vi "x410_test_fpga_simple.vi"() -> ()   [LabVIEW 2025]
doc: "this VI is the top level of the FPGA.\n\nsubVIs placed at this level:\nmust have fixed-sized arrays.\ncontaining a class input (control) must NOT be left unconnected.\n\nconditional symbols supported for ease-of-use in building variations of the image are documented in a comment section and should be kept up-to-date."
uses:
  Aqc_loop_states.ctl
  <instrlib>/_niInstr/DSP/v1/Shared/Public/IQ Gain.ctl
  FPGA/DataMode.ctl
  <vilib>/Platform/TimedLoop/XDataNode/timing_clust.ctl
  <vilib>/Platform/TimedLoop/XDataNode/nitl_modes.ctl
  <vilib>/Platform/TimedLoop/XDataNode/wakeup.ctl
  <vilib>/rvi/Emulation/niFpgaSctlEmulationGetInTimedLoop.vi
  <vilib>/rvi/Emulation/niFpgaEmulationReportErrorSimple.vi
  <vilib>/rvi/Emulation/niFpgaGetClockAttributes.vi
  <vilib>/rvi/Emulation/niFpgaCriticalErrorInLSC.vi
  <vilib>/rvi/Emulation/niFpgaEmulationIsFPGAContextNoSignature.vi
  <vilib>/rvi/DataTransferAndStorage/Container/Common/niFpgaContainerGetUniqueNameForEmu.vi
  <vilib>/rvi/Memory/Memory_Emulation/niFpgaMemoryEmulationCacheClearOnFirstRun.vi
  <vilib>/rvi/Memory/Memory_Emulation/nirvimemoryEmulationManagerCache_MakeExclusive.vi
  <vilib>/rvi/Memory/Memory_Emulation/niFpgaMemoryEmulationValidateCache.vi
  <vilib>/rvi/Memory/Memory_Emulation/nirvimemoryEmulationManagerCache_InsertValue.vi
  <vilib>/Utility/error.llb/Clear Errors.vi
  <vilib>/rvi/Memory/Memory_Emulation/nirvimemoryEmulationManagerCache_ReleaseExclusive.vi
  <vilib>/rvi/Memory/Memory_Emulation/nirvimemoryEmulationManagerCache_GetValue.vi
  <vilib>/rvi/Memory/Memory_Emulation/nirvimemoryEmulationManagerCache_SetValue.vi
  <vilib>/rvi/Emulation/niFpgaProcessEmulError.vi
  <vilib>/rvi/errors/niFpgaSetErrorForExecOnDevCompSimple.vi
  <vilib>/rvi/eio/common/nirviEmuReportErrorAndStop.vi
  <vilib>/rvi/FIFO/Fifo_Resource/nirvififoEmulationSetSize.vi
  <vilib>/rvi/FIFO/Fifo_Resource/nirviFifoEmulationQueueMgr.vi
  <instcachedir>/0/nirviFifoEmulationQueueMgr_E5CAEC123FF24DC58D834DCA3CDAA9B5.lvgen/nirviFifoEmulationQueueMgr_E5CAEC123FF24DC58D834DCA3CDAA9B5_017.vi
  <vilib>/rvi/FIFO/Fifo_Resource/nirvififoEmulationCreateLock.vi
  <vilib>/rvi/FIFO/Fifo_Resource/nirvififoEmulationObtainLock.vi
  <vilib>/rvi/FIFO/Fifo_Resource/nirvififoEmulationReleaseLock.vi
  <vilib>/rvi/occurrence/nirviWaitOnOccurrenceBase.vi
  <vilib>/rvi/errors/nirviReportUnexpectedCaseInternalError.vi
  <vilib>/rvi/errors/nirviReportUnexpectedCaseInternalError (U32).vi
  <instcachedir>/0/nirviFifoEmulationQueueMgr_E5CAEC123FF24DC58D834DCA3CDAA9B5.lvgen/nirviFifoEmulationQueueMgr_E5CAEC123FF24DC58D834DCA3CDAA9B5_016.vi
  <vilib>/rvi/FIFO/Fifo_Resource/nirvififoEmulationDetermineInputValidOut.vi
  <vilib>/rvi/interface/RandomDataEmulation/nirviRandomDataMultiElementFPGAFIFO.vi
  <instcachedir>/0/nirviRandomDataMultiElementFPGAFIFO_BE2FF10D3D6E420AB0291A02835C249E.lvgen/nirviRandomDataMultiElementFPGAFIFO_BE2FF10D3D6E420AB0291A02835C249E_001.vi
  <vilib>/rvi/interface/RandomDataEmulation/niFpgaRandomDataHandleErrors.vi
  <vilib>/Platform/TimedLoop/XDataNode/XDataNode.xnode
  <vilib>/rvi/DataTransferAndStorage/Container/XNode/niFpgaContainer.xnode
  <vilib>/rvi/DataTransferAndStorage/Register/Emulation/niFpgaRegisterEmulation.vi
  <vilib>/rvi/FIFO/Fifo_Resource/nirvififoEmulationRead.vi
  <vilib>/rvi/FIFO/Fifo_Resource/nirvififoEmulationWrite.vi
  <vilib>/rvi/interface/RandomDataEmulation/nirviRandomDataFpgaMultiElementTemplate.vi
  <vilib>/Platform/TimedLoop/XDataNode/XDNodeRunTimeDep.lvlib
  <instrlib>/niUSRP/Reference FPGA/Tx Core/niUSRP Tx Core v1 FPGA.lvclass
  <instrlib>/_niInstr/DSP/v1/Shared/niInstr DSP v1 Shared.lvlib
panel:
  in  "Host scale":u16
  in  "simulated phase":fxp<+,64,64>
  in  "Mode":T1
  in  "gain":T2={"gain I"=1.0, "gain Q"=1.0}
  out "loop states":T3
  in  "Record length":u16=4000 caption="Samples Per Trigger" min=1 step=1
  in  "Trigger Acquisition":bool
  in  "Acquisition running":bool
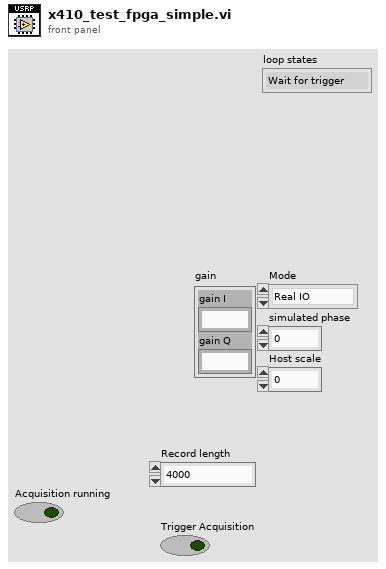
[diagram p1: front panel]
types:
  T1 = typedef "DataMode.ctl" = enum16{"Real IO", "Simulated"}
  T2 = typedef "niInstr DSP v1 Shared.lvlib/IQ Gain.ctl" = cluster{"gain I":fxp<+/-,24,3>, "gain Q":fxp<+/-,24,3>}
  T3 = typedef "Aqc_loop_states.ctl" = enum8{"Wait for trigger", "Acquisition", "Send record length", "Wait for output", "Quiet period"}
  T4 = typedef "XDNodeRunTimeDep.lvlib/timing_clust.ctl" = cluster{"Expected End [f-1]":u64, "Actual End [f-1]":u64, "Finished Late? [f-1]":bool, "Expected End [i-1]":u64, "Actual End [i-1]":u64, "Finished Late? [i-1]":bool, "Expected Start [i]":u64, "Actual Start [i]":u64, "Expected Start [f]":u64, "Actual Start [f]":u64, "Source Name":string, "Structure Name":string, "Period":i64, "Deadline":i64, "Offset":i64, "Start":i64, "Priority":i32, "Timeout":i32, "Mode":T5, "Wakeup Reason":T6, "Error":errorcluster, "Source Type":string, "Secondary Source Type":string, "Global End Time":u64, "Global Start Time":u64, "Frame Duration":u64, "Iteration Duration":u64, "Assigned CPU":i32, "I/O Scan Engine Mode":u32}
  T5 = typedef "XDNodeRunTimeDep.lvlib/nitl_modes.ctl" = enum32{"No Change", "Process missed periods, maintain original phase", "Discard missed periods, maintain original phase", "Process missed periods, ignore original phase", "Discard missed periods, ignore original phase"}
  T6 = typedef "XDNodeRunTimeDep.lvlib/wakeup.ctl" = enum32{"Normal", "Aborted", "Asynchronous wakeup", "Timing source error", "Timed loop error", "Timeout"}
  T7 = cluster{"I":fxp<+/-,18,1>, "Q":fxp<+/-,18,1>, "overflow":bool}[]
  T8 = typedef "niInstr DSP v1 Shared.lvlib/IQ Data.ctl" = cluster{"I":fxp<+/-,18,1>, "Q":fxp<+/-,18,1>, "overflow":bool}
  T9 = typedef "Array-18bit-8element.ctl" = fxp<+/-,18,1>[]
  T10 = cluster{"I":fxp<+/-,18,1>, "Q":fxp<+/-,18,1>, "overflow":bool}
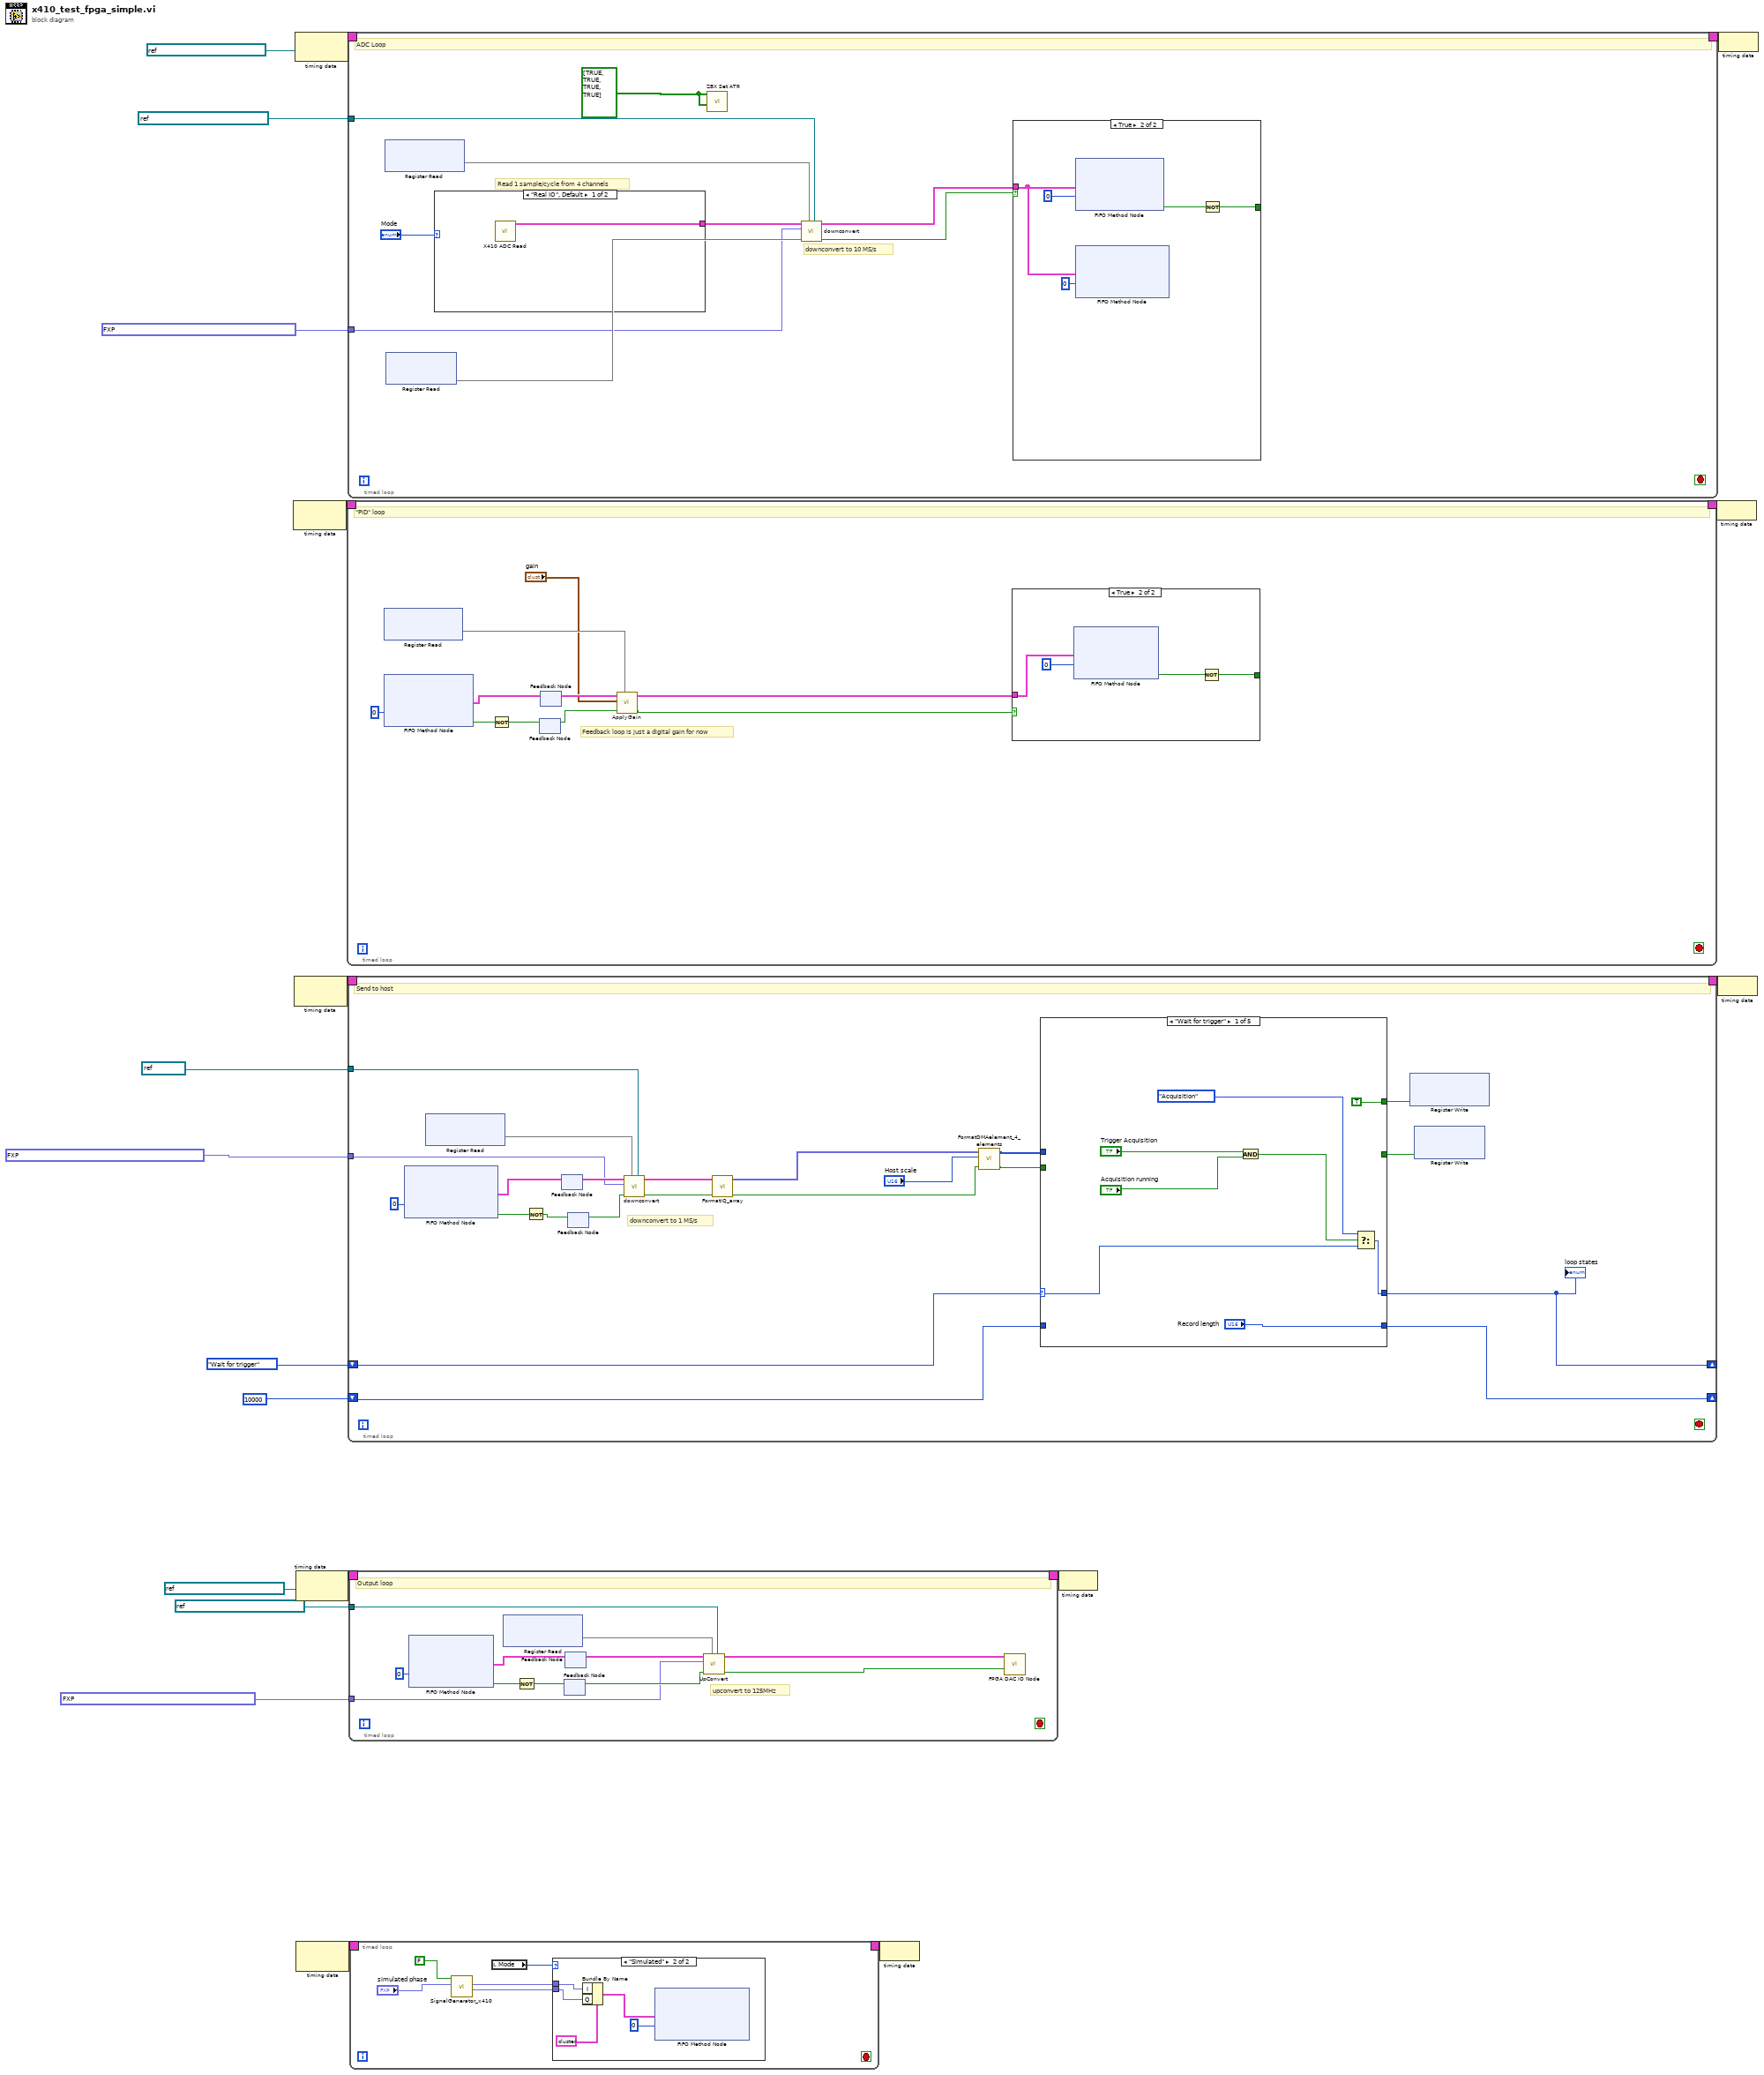
[diagram p0: block diagram]
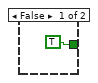
[diagram p3: hidden frame]
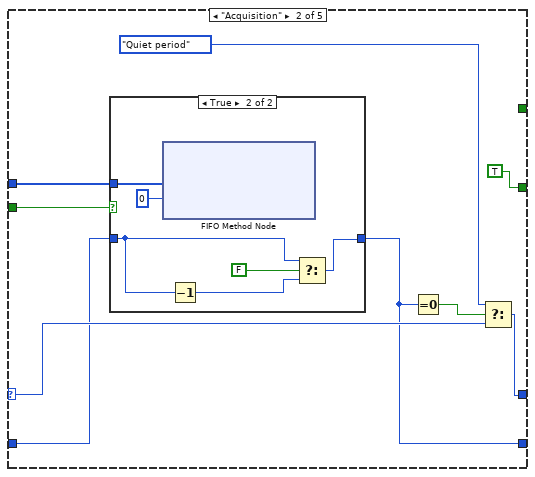
[diagram p4: hidden frame]
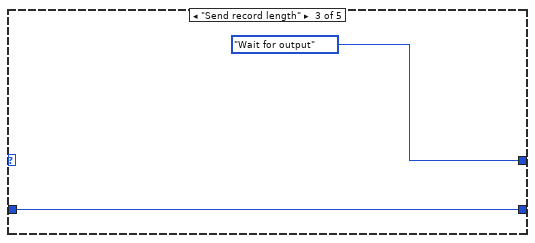
[diagram p6: hidden frame]
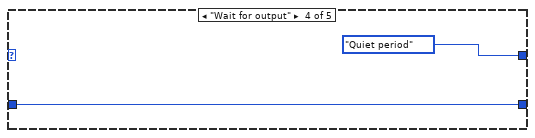
[diagram p7: hidden frame]
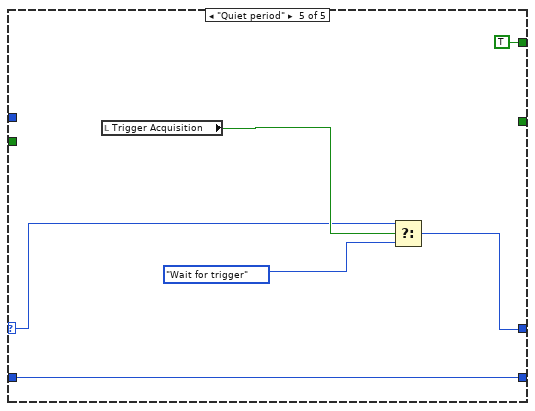
[diagram p8: hidden frame]
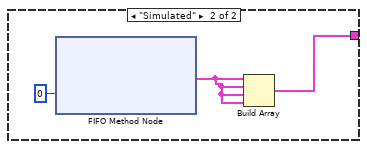
[diagram p9: hidden frame]
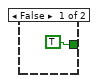
[diagram p10: hidden frame]
diagram:
  n1 = node-c288() -> (w11:T4)  [unwired: 1 in]
  n2 = node-c288() -> (w17:T4)  [unwired: 1 in]
  n3 = node-c288(refnum<k21> "Daughterboard 0\\Data Clock" ("Source Name")) -> (w20:T4)
  n4 = node-c288(refnum<k21> "Daughterboard 0\\Data Clock" ("Source Name")) -> (w7:T4)
  n5 = node-c288() -> (w2:T4)  [unwired: 1 in]
  n6 = timed-loop "Acquisition Loop" {
    timing: w11 -> [_]
    timing-out: [_] -> w10
    stop <- _ stop-if-true
    # "Feedback loop is just a digital gain for now"
    # "\"PID\" loop"
    n7 = xnode "Register Read"() -> ("Data"=w25)  [unwired: 1 in, 1 out]
    n8 = xnode ("FIFO Method Node")("Timeout"=0) -> ("Element"=w29:T7, "Timed Out?"=w30:bool)  [unwired: 1 in, 1 out]
    n9 = Not(x=w30) -> (.not. x?=w27:bool)
    n10 = feedback #1() -> (w26:bool)  [unwired: 1 in]
    n11 = feedback-in #1(w27) -> ()
    n12 = feedback #2() -> (w28:T7)  [unwired: 1 in]
    n13 = feedback-in #2(w29) -> ()
    n14 = call "ApplyGain.vi"("reset"=w25, "input valid"=w26, "gain"="gain", "data in"=w28) -> ("output valid"=w23:bool, "data out"=w22:T8[])  [unwired: 6 in]
    n15 = case shown="True" w23 {
      tunnel: [TRUE ("Timed Out?") w33] -> _
      tunnel: w22 -> [_ w32]
      frame False {
      }
      frame True {
        n16 = xnode ("FIFO Method Node")("Element"=w32, "Timeout"=0) -> ("Timed Out?"=w34:bool)  [unwired: 1 in, 1 out]
        n17 = Not(x=w34) -> (.not. x?=w33:bool)
      }
    }
  }
  n18 = timed-loop "Acquisition Loop" {
    timing: w17 -> [_]
    timing-out: [_] -> w16
    shift-right: [w55] -> _
    shift-left: u16 10000 ("Record length") -> [w53]
    shift-right: [w56] -> _
    shift-left: Aqc_loop_states."Wait for trigger" ("loop states") -> [w54]
    tunnel: refnum<k21> "20MHz" ("clock x2") -> [w44]
    tunnel: fxp<+,48,1> 0.10000000000000142 ("output sample rate") -> [w42]
    stop <- _ stop-if-true
    # "downconvert to 1 MS/s"
    # "Send to host"
    n19 = xnode ("FIFO Method Node")("Timeout"=0) -> ("Element"=w49:T7, "Timed Out?"=w51:bool)  [unwired: 1 in, 1 out]
    n20 = xnode "Register Read"() -> ("Data"=w43)  [unwired: 1 in, 1 out]
    n21 = Not(x=w51) -> (.not. x?=w50:bool)
    n22 = feedback #3() -> (w46:T7)  [unwired: 1 in]
    n23 = feedback-in #3(w49) -> ()
    n24 = feedback-in #4(w50) -> ()
    n25 = feedback #4() -> (w45:bool)  [unwired: 1 in]
    n26 = call "downconvert.vi"("clock x2"=w44, "reset"=w43, "input valid"=w45, "output sample rate"=w42, "data in"=w46) -> ("output valid"=w40:bool, "data out"=w41:T8[])  [unwired: 5 in]
    n27 = call "FormatIQ_array"("valid in"=w40, "data in"=w41) -> ("valid out"=w38:bool, "Array"=w39:T9)  [unwired: 8 in]
    n28 = call "FormatDMAelement_4_elements.vi"("valid in"=w38, "factor"="Host scale", "Array"=w39) -> ("valid out"=w57:bool, "Values"=w58:u64[])  [unwired: 7 in]
    n29 = case shown="\"Wait for trigger\"" w54 {
      selector: w54 -> [w67 w76 _ _ w90]
      tunnel: w53 -> [_ w73 w85 w87 w91]
      tunnel: [w66 w75 Aqc_loop_states."Wait for output" ("loop states") Aqc_loop_states."Quiet period" ("loop states") w92] -> w56
      tunnel: ["Record length" w70 w85 w87 w91] -> w55
      tunnel: w58 -> [_ w71 _ _ _]
      tunnel: w57 -> [_ w72 _ _ _]
      tunnel: [_ TRUE _ _ _] -> w48
      tunnel: [TRUE _ _ _ TRUE] -> w47
      frame "Wait for trigger" {
        n30 = And(x="Trigger Acquisition", y="Acquisition running") -> (x .and. y?=w61:bool)
        n31 = Select(t=Aqc_loop_states."Acquisition" ("loop states"), s=w61, f=w67) -> (s? t:f=w66:T3)
      }
      frame "Acquisition" {
        n32 = case shown="True" w72 {
          tunnel: w71 -> [_ w83]
          tunnel: [w77 w81] -> w70
          tunnel: w73 -> [w77 w79]
          frame False {
          }
          frame True {
            n33 = xnode ("FIFO Method Node")("Element"=w83, "Timeout"=0) -> ()  [unwired: 1 in, 2 out]
            n34 = Decrement(x=w79) -> (x-1=w80:u16)
            n35 = Select(t=w79, s=FALSE, f=w80) -> (s? t:f=w81:u16)
          }
        }
        n36 = Equal To 0?(x=w70) -> (x = 0?=w74:bool)
        n37 = Select(t=Aqc_loop_states."Quiet period" ("loop states"), s=w74, f=w76) -> (s? t:f=w75:T3)
      }
      frame "Send record length" {
      }
      frame "Wait for output" {
      }
      frame "Quiet period" {
        n38 = local read "Trigger Acquisition"() -> (w93:bool)
        n39 = Select(t=w90, s=w93, f=Aqc_loop_states."Wait for trigger" ("loop states")) -> (s? t:f=w92:T3)
      }
    }
    "loop states" <- w56
    n40 = xnode "Register Write"("Data"=w47) -> ()  [unwired: 1 in, 1 out]
    n41 = xnode "Register Write"("Data"=w48) -> ()  [unwired: 1 in, 1 out]
  }
  n42 = timed-loop "Acquisition Loop" {
    timing: w20 -> [_]
    timing-out: [_] -> w19
    tunnel: fxp<+,48,1> 0.0799999999999983 ("output sample rate") -> [w103]
    tunnel: refnum<k21> "Daughterboard 0\\Data Clock x2" ("clock x2") -> [w97]
    stop <- _ stop-if-true
    w100 = bool[] [TRUE, TRUE, TRUE, TRUE] ("DB 0")
    # "Read 1 sample/cycle from 4 channels"
    # "downconvert to 10 MS/s"
    # "ADC Loop"
    n43 = xnode "Register Read"() -> ("Data"=w101)  [unwired: 1 in, 1 out]
    n44 = xnode "Register Read"() -> ("Data"=w104)  [unwired: 1 in, 1 out]
    n45 = case shown="\"Real IO\", Default" "Mode" {
      tunnel: [w105 w107] -> w102
      frame "Real IO", Default {
        n46 = call <instrlib>:"X410 ADC Read.vi"() -> ("Data out"=w105:T8[])  [unwired: 11 in]
      }
      frame "Simulated" {
        n47 = xnode ("FIFO Method Node")("Timeout"=0) -> ("Element"=w108:T10)  [unwired: 1 in, 2 out]
        n48 = Build Array(w108, w108, w108, w108) -> (w107:T7)
      }
    }
    n49 = call <instrlib>:"ZBX Set ATR.vi"("DB 1"=w100, "DB 0"=w100) -> ()  [unwired: 10 in]
    n50 = call "downconvert.vi"("clock x2"=w97, "reset"=w101, "input valid"=w104, "output sample rate"=w103, "data in"=w102) -> ("output valid"=w98:bool, "data out"=w99:T8[])  [unwired: 5 in]
    n51 = case shown="True" w98 {
      tunnel: w99 -> [_ w111]
      tunnel: [TRUE ("Timed Out?") w112] -> _
      frame False {
      }
      frame True {
        n52 = xnode ("FIFO Method Node")("Element"=w111, "Timeout"=0) -> ("Timed Out?"=w113:bool)  [unwired: 1 in, 1 out]
        n53 = xnode ("FIFO Method Node")("Element"=w111, "Timeout"=0) -> ()  [unwired: 1 in, 2 out]
        n54 = Not(x=w113) -> (.not. x?=w112:bool)
      }
    }
  }
  n55 = timed-loop "Acquisition Loop" {
    timing: w7 -> [_]
    timing-out: [_] -> w6
    tunnel: refnum<k21> "Daughterboard 0\\Data Clock x2" ("clock x2") -> [w118]
    tunnel: fxp<+,48,1> 0.0799999999999983 ("output sample rate") -> [w117]
    stop <- _ stop-if-true
    # "upconvert to 125MHz"
    # "Output loop"
    n56 = xnode ("FIFO Method Node")("Timeout"=0) -> ("Element"=w126:T7, "Timed Out?"=w127:bool)  [unwired: 1 in, 1 out]
    n57 = xnode "Register Read"() -> ("Data"=w123)  [unwired: 1 in, 1 out]
    n58 = Not(x=w127) -> (.not. x?=w125:bool)
    n59 = feedback #5() -> (w122:bool)  [unwired: 1 in]
    n60 = feedback-in #5(w125) -> ()
    n61 = feedback #6() -> (w120:T7)  [unwired: 1 in]
    n62 = feedback-in #6(w126) -> ()
    n63 = call "UpConvert.vi"("clock x2"=w118, "reset"=w123, "input valid"=w122, "output sample rate"=w117, "data in"=w120) -> ("output valid"=w121:bool, "data out"=w119:T8[])  [unwired: 5 in]
    n64 = call <instrlib>:"FPGA DAC IO Node.vi"("data"=w119, "input valid"=w121) -> ()  [unwired: 14 in]
  }
  n65 = timed-loop {
    timing: w2 -> [_]
    timing-out: [_] -> w1
    stop <- _ stop-if-true
    n66 = call "SignalGenerator_x410.vi"("phase"="simulated phase", "Reset"=FALSE) -> ("Cos"=w130:fxp<+/-,18,1>, "Sin"=w131:fxp<+/-,18,1>)  [unwired: 7 in, 1 out]
    n67 = local read "Mode"() -> (w132:T1)
    n68 = case shown="\"Simulated\"" w132 {
      tunnel: w131 -> [_ w137]
      tunnel: w130 -> [_ w136]
      frame "Real IO", Default {
      }
      frame "Simulated" {
        n69 = Bundle By Name(cluster=T10 {"I"=0.0, "Q"=0.0, "overflow"=FALSE} ("Element"), "I"=w137, "Q"=w136) -> (w135:T10)
        n70 = xnode ("FIFO Method Node")("Element"=w135, "Timeout"=0) -> ()  [unwired: 1 in, 2 out]
      }
    }
  }
  n71 = node-c288(w1) -> ()
  n72 = node-c288(w6) -> ()
  n73 = node-c288(w10) -> ()
  n74 = node-c288(w16) -> ()
  n75 = node-c288(w19) -> ()
